vi "HeaderAction.vi"(0 "InstrClass":refnum<class "ESP301.lvclass"> caption="DNL_LabVIEW Object in", 11 "error in (no error)":errorcluster caption="entrée d'erreur (pas d'erreur)") -> (4 "InstrClassOut":refnum<class "ESP301.lvclass"> caption="DNL_LabVIEW Object out", 6 "DataNames":string[](array[string]), 8 "Instr Name":string, 10 "HeaderString":string, 13 "ArrDisplayNames":string[](array[string]), 14 "DisplayNames":string[](array[string]), 15 "error out":errorcluster caption="sortie d'erreur")   [LabVIEW 2019, in "ESP301.lvclass"]
uses:
  ESP301.lvclass
  C:/Programmes Labview/LabScanV1A/DevicesClass/BaseDevice/BaseDevice.lvclass
  ESP301.lvclass/ESP301.ctl
  ESP301_Func.ctl
  BaseDevice/BaseDevice.lvclass
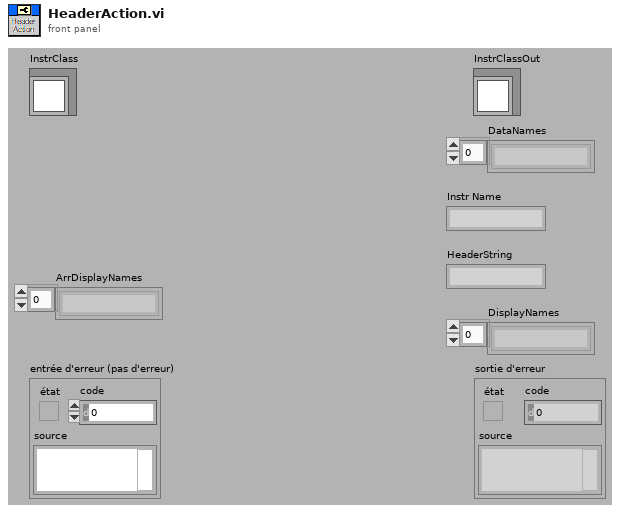
[diagram p1: front panel]
types:
  T1 = typedef "ESP301.lvclass/ESP301_Func.ctl" = enum16{"Position (mm)", "MirrorSlide (pos)"}
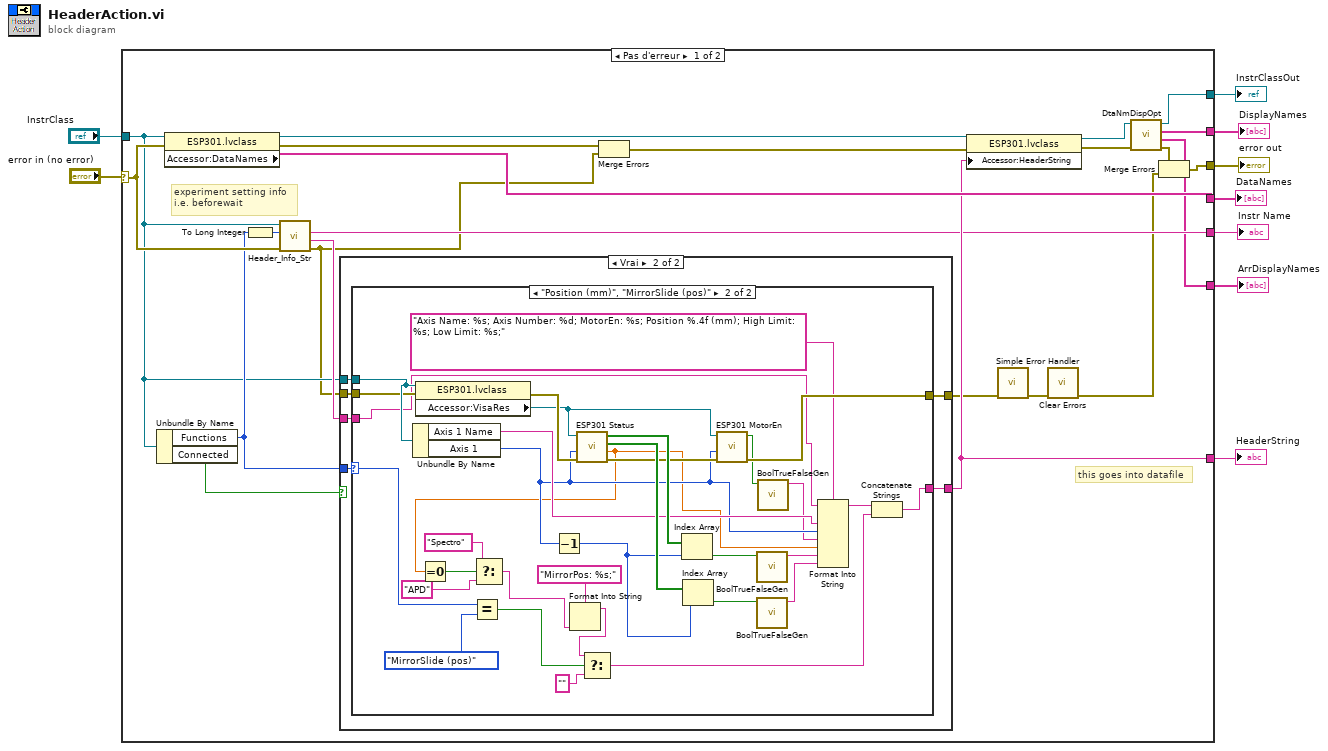
[diagram p0: block diagram]
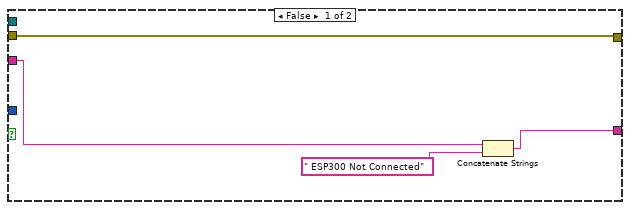
[diagram p2: hidden frame]
diagram:
  n1 = case shown="Pas d'erreur" "error in (no error)" {
    selector: "error in (no error)" -> [w21 w78]
    tunnel: [w29 _] -> w8
    tunnel: [w32 _] -> w7
    tunnel: "InstrClass" -> [w16 w79]
    tunnel: [w14 w78] -> w5
    tunnel: [w26 w79] -> w3
    tunnel: [w23 _] -> w4
    tunnel: [w24 _] -> w2
    tunnel: [w17 _] -> w1
    frame No Error {
      # "this goes into datafile"
      # "experiment setting info\ni.e. beforewait"
      n2 = Unbundle By Name(w16) -> ("Functions"=w19:T1, "Connected"=w10:bool)
      n3 = property class="ESP301.lvclass"(reference=w16, error in=w21) -> (reference out=w31:refnum<class "ESP301.lvclass">, error out=w30:errorcluster, "Accessor:DataNames"=w32:string[])
      n4 = To Long Integer(number=w19) -> (32bit integer=w18:i32)
      n5 = call-dynamic "Header_Info_Str.vi"("error in (no error)"=w21, "Functions"=w18, "DefaultDev in"=w16) -> ("error out"=w15:errorcluster, "HdrInfoStr"=w22:string, "InstrumentName"=w23:string)  [unwired: 5 in, 1 out]
      n6 = case shown="Vrai" w10 {
        tunnel: [w34 w42] -> w29
        tunnel: w22 -> [w35 w41]
        tunnel: w19 -> [_ w40]
        tunnel: w16 -> [_ w39]
        tunnel: w15 -> [w33 w38]
        tunnel: [w33 w37] -> w13
        frame False {
          n7 = Concatenate Strings(w35, " ESP300 Not Connected" ("chaîne")) -> (w34:string)
        }
        frame True {
          n8 = case shown="\"Position (mm)\", \"MirrorSlide (pos)\"" w40 {
            selector: w40 -> [_ w58]
            tunnel: [w43 w47] -> w42
            tunnel: w41 -> [w43 w45]
            tunnel: w39 -> [_ w71]
            tunnel: w38 -> [w44 w70]
            tunnel: [w44 w69] -> w37
            frame Default {
            }
            frame "Position (mm)", "MirrorSlide (pos)" {
              n9 = Unbundle By Name(w71) -> ("Axis 1 Name"=w66:string, "Axis 1"=w62:u8)
              n10 = property class="ESP301.lvclass"(reference=w71, error in=w70) -> (error out=w77:errorcluster, "Accessor:VisaRes"=w73:refnum<visa-resource-name>)  [unwired: 1 out]
              n11 = Equal?(x=w58, y=ESP301_Func."MirrorSlide (pos)") -> (x = y?=w56:bool)
              n12 = Decrement(x=w62) -> (x-1=w72:u8)
              n13 = call <userlib>:"ESP301 Status.vi"("error in"=w77, "Axis"=w62, "VISA Rsrc"=w73) -> ("error out"=w74:errorcluster, "Position"=w54:dbl, "Low Limit"=w75:bool[], "High Limit"=w76:bool[])  [unwired: 5 in]
              n14 = Equal To 0?(x=w54) -> (x = 0?=w53:bool)
              n15 = Select(t="Spectro", s=w53, f="APD") -> (s? t:f=w49:string)
              n16 = Format Into String(format string="MirrorPos: %s;" ("chaîne de format"), w49) -> (resulting string=w48:string)  [unwired: 2 in, 1 out]
              n17 = Select(t=w48, s=w56, f="") -> (s? t:f=w46:string)
              n18 = Index Array(array=w76, index=w72) -> (element=w65:bool)
              n19 = Index Array(array=w75, index=w72) -> (element=w67:bool)
              n20 = call <userlib>:"ESP301 MotorEn.vi"("error in"=w74, "Axis"=w62, "VISA Rsrc"=w73) -> ("error out"=w69:errorcluster, "MotorEnOut"=w61:bool)  [unwired: 7 in]
              n21 = call <userlib>:"BoolTrueFalseGen.vi"("Bool"=w65) -> ("TrueFalse"=w64:string)  [unwired: 8 in, 1 out]
              n22 = call <userlib>:"BoolTrueFalseGen.vi"("Bool"=w67) -> ("TrueFalse"=w63:string)  [unwired: 8 in, 1 out]
              n23 = call <userlib>:"BoolTrueFalseGen.vi"("Bool"=w61) -> ("TrueFalse"=w60:string)  [unwired: 8 in, 1 out]
              n24 = Format Into String(format string="Axis Name: %s; Axis Number: %d; MotorEn: %s; Position %.4f (mm); High Limit: %s; Low Limit: %s;" ("chaîne de format"), initial string=w45, w66, w62, w60, w54, w64, w63) -> (resulting string=w59:string)  [unwired: 1 in, 1 out]
              n25 = Concatenate Strings(w59, w46) -> (w47:string)
            }
          }
        }
      }
      n26 = Merge Errors(w30, w15) -> (w20:errorcluster)
      n27 = property class="ESP301.lvclass"(reference=w31, error in=w20, "Accessor:HeaderString"=w29) -> (reference out=w25:refnum<class "ESP301.lvclass">, error out=w28:errorcluster)
      n28 = call <vilib>:"Simple Error Handler.vi"("error in (no error)"=w13) -> ("error out"=w12:errorcluster)  [unwired: 4 in, 4 out]
      n29 = call <vilib>:"Clear Errors.vi"("error in (no error)"=w12) -> ("error out"=w11:errorcluster)  [unwired: 5 in, 1 out]
      n30 = call "DtaNmDispOpt.vi"("error in (no error)"=w28, "BaseDevice en entrée"=w25) -> ("error out"=w27:errorcluster, "ArrDisplayNames"=w17:string[], "DisplayNames"=w24:string[], "BaseDevice en sortie"=w26:refnum<class "ESP301.lvclass">)  [unwired: 6 in]
      n31 = Merge Errors(w27, w11) -> (w14:errorcluster)
    }
    frame Error {
    }
  }
  "error out" <- w5
  "InstrClassOut" <- w3
  "DataNames" <- w7
  "HeaderString" <- w8
  "Instr Name" <- w4
  "DisplayNames" <- w2
  "ArrDisplayNames" <- w1
